vi "Straight-Line Equation.vi"() -> ()   [LabVIEW 2026]
doc: "Descrizione VI"
panel:
  in  "Measurement 2":enum16{"tipo2", "tipo 1"}(ring)
  in  "Measurement Type":T1(ring)
  out "Average":dbl
  in  "X5":dbl
  in  "X4":dbl
  in  "X3":dbl
  in  "X2":dbl
  in  "X1":dbl
  in  "Slope (m)":dbl
  in  "X":dbl
  out "y":dbl
  in  "Y-Intercept (b)":dbl
  # "Comment"
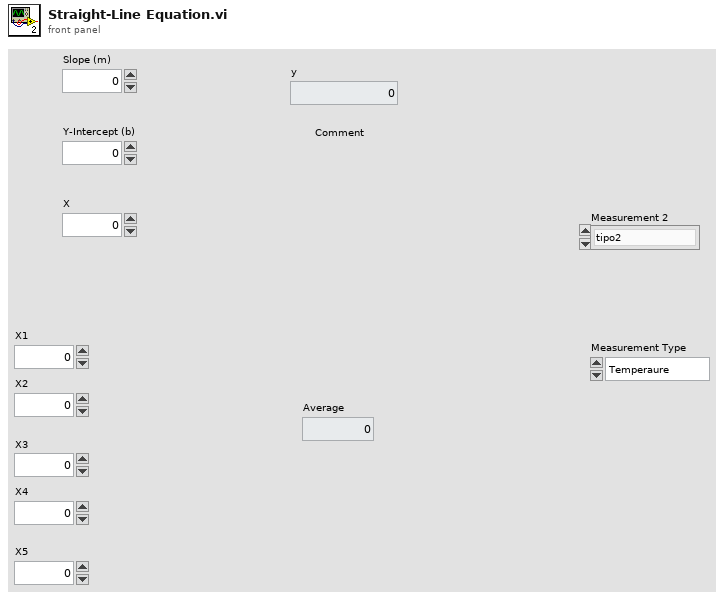
[diagram p1: front panel]
types:
  T1 = enum16{"Temperaure", "Pressure", "Resistance", "Voltage"}
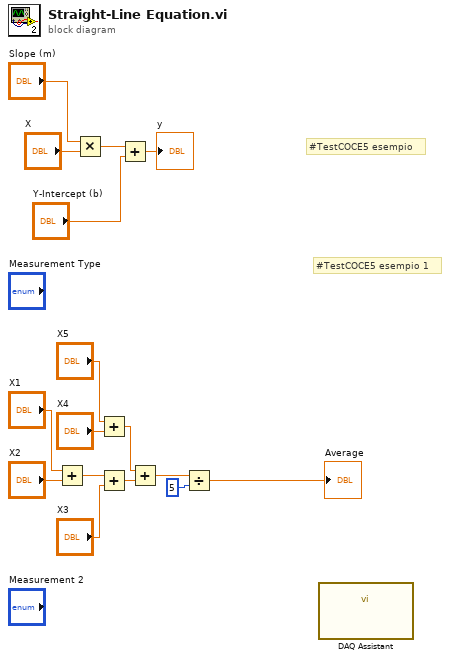
[diagram p0: block diagram]
diagram:
  # "#TestCOCE5 esempio 1"
  # "#TestCOCE5 esempio"
  n1 = Add(x="X1", y="X2") -> (x+y=w9:dbl)
  n2 = Multiply(x="Slope (m)", y="X") -> (x*y=w14:dbl)
  n3 = Add(x="X5", y="X4") -> (x+y=w6:dbl)
  n4 = Add(x=w9, y="X3") -> (x+y=w5:dbl)
  n5 = Add(x=w14, y="Y-Intercept (b)") -> (x+y=→"y":dbl)
  n6 = Add(x=w6, y=w5) -> (x+y=w2:dbl)
  n7 = Divide(x=w2, y=5) -> (x/y=→"Average":dbl)
  n8 = call "DAQ Assistant"() -> ()  [unwired: 12 in]
